vi "from string.vi"(8 "error in":errorcluster, 9 "data":string, 10 "version":string, 11 "DIO Channel configuration in":refnum<class "Digital IO Channel configuration.lvclass">) -> (0 "error out":errorcluster, 3 "DIO Channel configuration out":refnum<class "Digital IO Channel configuration.lvclass">)   [LabVIEW 2025, in "Digital IO.lvlib" / "Digital IO Channel configuration.lvclass"]
doc: "Provides an interface for loading a module configuration from a file or other serialized data source. It is recommended that all children of this class store data in two sets--data required for its own initialization, and any data required for parent initialization--and that each implementation uses the <b>Call Parent Method</b> primitive to de-serialize parent information.Copyright 2017 National Instruments Corporation\n\nLicensed under the Apache License, Version 2.0 (the \"License\"); you may not use this file except in compliance with the License. You may obtain a copy of the License at http://www.apache.org/licenses/LICENSE-2.0\nUnless required by applicable law or agreed to in writing, software distributed under the License is distributed on an \"AS IS\" BASIS, WITHOUT WARRANTIES OR CONDITIONS OF ANY KIND, either express or implied. See the License for the specific language governing permissions and limitations under the License."
uses:
  Digital IO Channel configuration.lvclass
  DIO Channel Setting.ctl
  Digital IO Channel configuration.lvclass/Digital IO Channel configuration.ctl
  Users/Public/Documents/Sandia National Labs/TSS Plugin/Abstract Engine.lvlibp/Channel configuration/Channel configuration.lvclass
  Users/Public/Documents/Sandia National Labs/TSS Plugin/CEF.lvlibp/serializable configuration/CEF_serializable configuration.lvclass
  Users/Public/Documents/Sandia National Labs/TSS Plugin/CEF.lvlibp
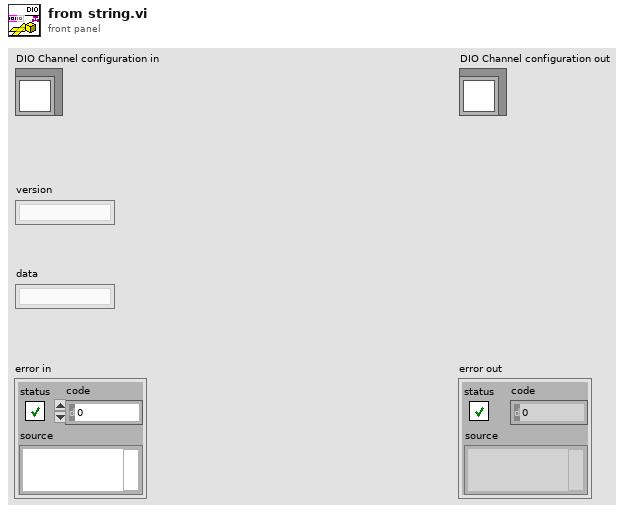
[diagram p1: front panel]
types:
  T1 = typedef "Digital IO.lvlib/Digital IO Channel configuration.lvclass/DIO Channel Setting.ctl" = cluster{"Connection":string}
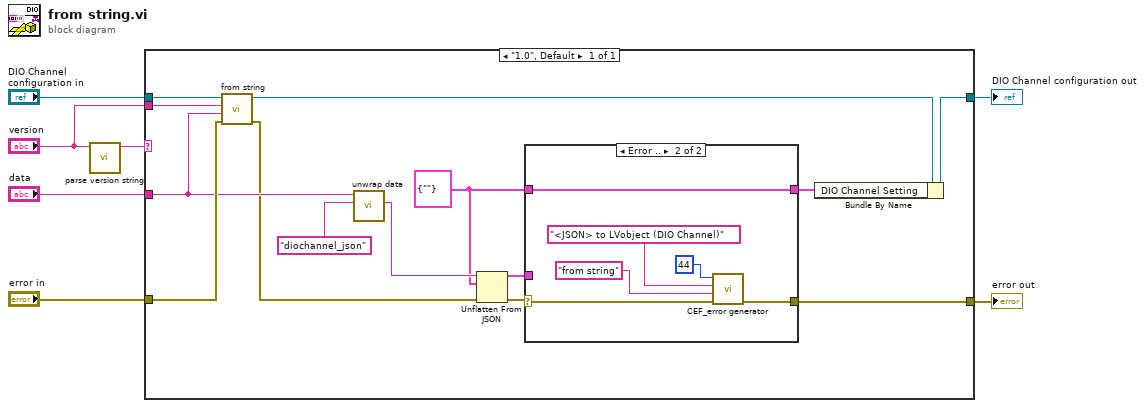
[diagram p0: block diagram]
diagram:
  n1 = call "parse version string.vi"("full version"="version") -> ("major.minor version"=w2:string)  [unwired: 7 in, 3 out]
  n2 = case shown="\"1.0\", Default" w2 {
    tunnel: "DIO Channel configuration in" -> [w21]
    tunnel: [w17] -> w6
    tunnel: "data" -> [w16]
    tunnel: "error in" -> [w18]
    tunnel: [w9] -> w5
    tunnel: "version" -> [w15]
    frame "1.0", Default {
      w10 = T1 {"Connection"=""} ("Setting")
      n3 = call-parent "from string.vi"("error in"=w18, "data"=w16, "version"=w15, "Channel configuration"=w21) -> ("error out"=w12:errorcluster, "Channel configuration out"=w20:refnum<class "Digital IO Channel configuration.lvclass">)  [unwired: 6 in]
      n4 = call "unwrap data.vi"("identifier"="diochannel_json" ("additional identifier"), "data to unwrap"=w16) -> ("unwrapped data"=w11:string)  [unwired: 8 in, 1 out]
      n5 = Unflatten From JSON(JSON string=w11, type and defaults=w10, error in (no error)=w12) -> (value=w14:T1, error out=w13:errorcluster)  [unwired: 4 in]
      n6 = case shown="Error .." w13 {
        selector: w13 -> [w22 w26]
        tunnel: w14 -> [w23 _]
        tunnel: [w23 w25] -> w8
        tunnel: w10 -> [_ w25]
        tunnel: [w22 w24] -> w9
        frame No Error {
        }
        frame Error {
          n7 = call "CEF_error generator.vi"("error in"=w26, "source"="from string" ("message"), "append error message"="<JSON> to LVobject (DIO Channel)" ("message"), "error code (0)"=44) -> ("error out"=w24:errorcluster)  [unwired: 5 in]
        }
      }
      n8 = Bundle By Name(cluster=w20, "DIO Channel Setting"=w8) -> (w17:refnum<class "Digital IO Channel configuration.lvclass">)
    }
  }
  "error out" <- w5
  "DIO Channel configuration out" <- w6
